vi "Z Aux Search Ethlist.vi"(8 "error in (no error)":errorcluster caption="错误输入（无错误）", 9 "uims":u32, 10 "addrbufflength":u32, 11 "ipaddrlist":string) -> (0 "error out":errorcluster caption="错误输出", 2 "function return":i32, 3 "ipaddrlist out":string)   [LabVIEW 2015, in "zauxdll.lvlib"]
doc: "int32 __stdcall ZAux_SearchEthlist(char *ipaddrlist, uint32 addrbufflength, uint32 uims);"
uses:
  zauxdll.lvlib
  Radar - 2015 32bit_autoqueue_angle_0319/zauxdll-2014/zauxdll.dll
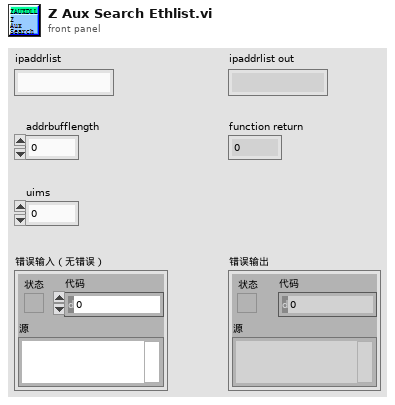
[diagram p1: front panel]
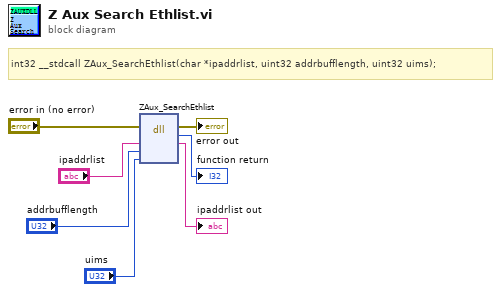
[diagram p0: block diagram]
diagram:
  # "int32 __stdcall ZAux_SearchEthlist(char *ipaddrlist, uint32 addrbufflength, uint32 uims);"
  n1 = dll-call lib="D:/vicomm case/cub/0717/Radar - 2015 32bit_autoqueue_angle_0319/zauxdll-2014/zauxdll.*" fn="ZAux_SearchEthlist"(error in="error in (no error)", "ipaddrlist"="ipaddrlist", "addrbufflength"="addrbufflength", "uims"="uims") -> (error out=→"error out":errorcluster, →"function return":i32, "ipaddrlist"=→"ipaddrlist out":string)  [unwired: 4 in, 1 out]
